vi "Controls_Get references.vi"(8 "error in (no error)":errorcluster, 11 "VI in":refnum<vi>) -> (0 "error out":errorcluster, 2 "Labels of Controls":string[](array[string]), 3 "References of Controls":refnum<vi>[](array[refnum]))   [LabVIEW 2016]
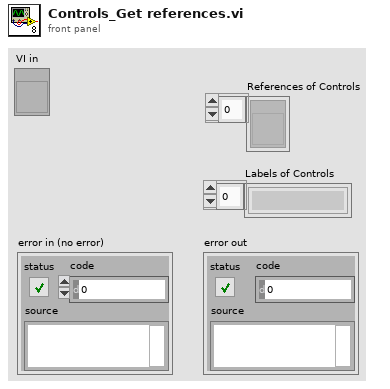
[diagram p1: front panel]
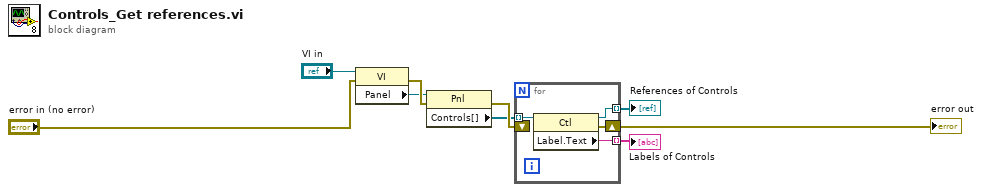
[diagram p0: block diagram]
diagram:
  n1 = property class="VI"(reference="VI in", error in="error in (no error)") -> (error out=w5:errorcluster, "Panel"=w2:refnum<vi>)  [unwired: 1 out]
  n2 = property class="Pnl"(reference=w2, error in=w5) -> (error out=w4:errorcluster, "Controls[]"=w3:refnum<vi>[])  [unwired: 1 out]
  n3 = for {
    tunnel: w3 -> [w13] mode=indexing
    shift-right: [w10] -> w7
    shift-left: w4 -> [_]
    tunnel: [w12] -> w9 mode=indexing
    tunnel: [w11] -> w8 mode=indexing
    n4 = property class="Ctl"(reference=w13) -> (reference out=w11:refnum<vi>, error out=w10:errorcluster, "Label.Text"=w12:string)  [unwired: 1 in]
  }
  "Labels of Controls" <- w9
  "References of Controls" <- w8
  "error out" <- w7
